vi "Read Voltage Setpoint.vi"   [LabVIEW 2023, in "Voltage Control.lvclass"]
uses:
  Voltage Control.lvclass
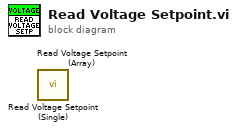
[diagram p0: block diagram]
diagram:
  n1 = call "Read Voltage Setpoint (Single).vi"() -> ()  [unwired: 8 in, 4 out]
  n2 = call "Read Voltage Setpoint (Array).vi"() -> ()  [unwired: 8 in, 4 out]
